vi "niFpgaButterflyTemp_2Pipe.vi"(0 "x_r":fxp<+/-,16,1>, 1 "mult output type":fxp<+/-,18,2>, 2 "bf bullet type":fxp<+/-,32,16> format="%.21g", 5 "x_i":fxp<+/-,16,1>, 7 "y_r":fxp<+/-,16,1>, 9 "y_i":fxp<+/-,16,1>, 12 "tf_r":fxp<+/-,16,1>, 13 "tf_i":fxp<+/-,16,1>, 14 "first stage":bool) -> (4 "x_out_r":fxp<+/-,16,1>, 6 "x_out_i":fxp<+/-,16,1>, 8 "y_out_r":fxp<+/-,16,1>, 10 "y_out_i":fxp<+/-,16,1>)   [LabVIEW 2017]
uses:
  <vilib>/rvi/FXPMathLib/FxpMul/XNode/nifxpmath_Multiplier.xnode
  <vilib>/rvi/FXPMathLib/sim/FxpSim.dll
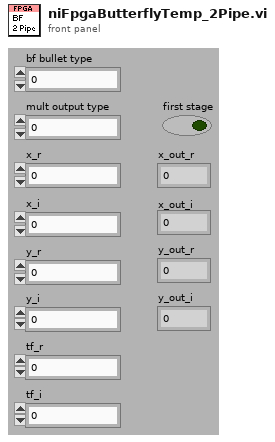
[diagram p1: front panel]
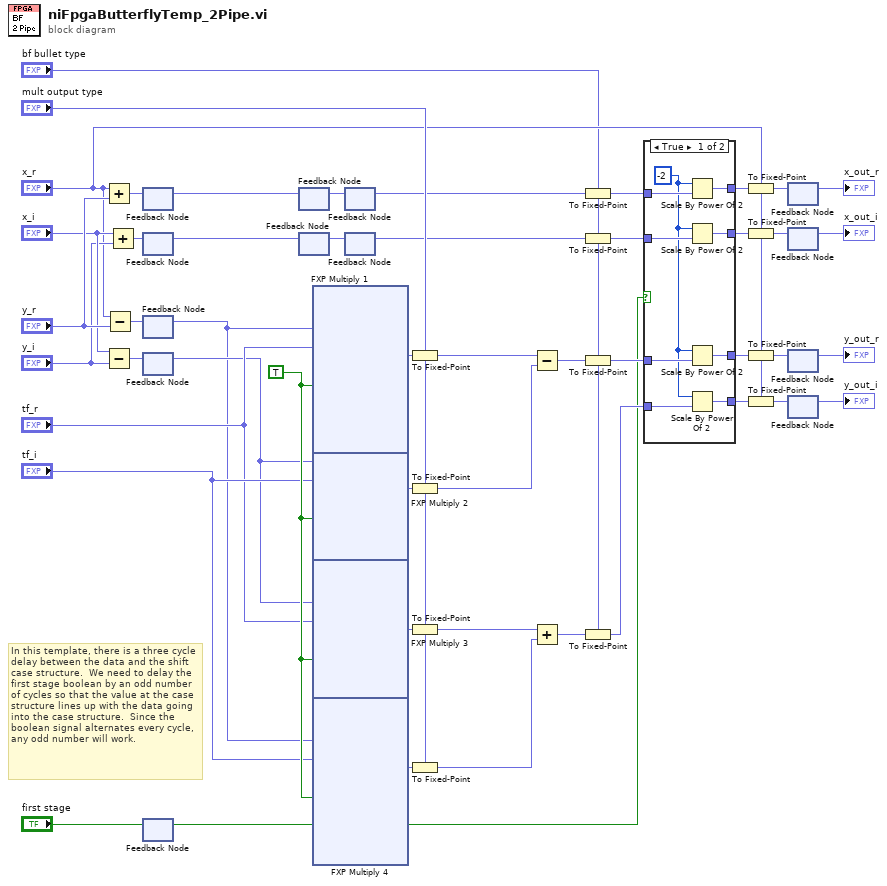
[diagram p0: block diagram]
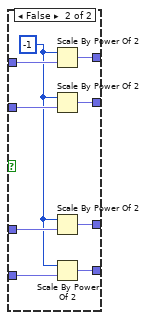
[diagram p2: hidden frame]
diagram:
  w40 = TRUE ("input valid")
  # "In this template, there is a three cycle delay between the data and the shift case structure.  We need to delay the first stage boolean by an odd number of cycles so that the value at the case structure lines up with the data going into the case structure.  Since the boolean signal alternates every cycle, any odd number will work."
  n1 = Add(x="x_r", y="y_r") -> (x+y=w37:fxp<+/-,17,2>)
  n2 = Subtract(x="x_i", y="y_i") -> (x-y=w48:fxp<+/-,17,2>)
  n3 = Subtract(x="x_r", y="y_r") -> (x-y=w49:fxp<+/-,17,2>)
  n4 = Add(x="x_i", y="y_i") -> (x+y=w16:fxp<+/-,17,2>)
  n5 = feedback-in #1(w37) -> ()
  n6 = feedback #1() -> (w20:fxp<+/-,17,2>)  [unwired: 1 out]
  n7 = feedback-in #2(w16) -> ()
  n8 = feedback #2() -> (w18:fxp<+/-,17,2>)  [unwired: 1 out]
  n9 = feedback-in #3(w49) -> ()
  n10 = feedback #3() -> (w14:fxp<+/-,17,2>)  [unwired: 1 out]
  n11 = feedback-in #4(w48) -> ()
  n12 = feedback #4() -> (w15:fxp<+/-,17,2>)  [unwired: 1 out]
  n13 = feedback-in #5("first stage") -> ()
  n14 = feedback #5() -> (w2:bool)  [unwired: 1 out]
  n15 = feedback-in #6(w20) -> ()
  n16 = feedback #6() -> (w19:fxp<+/-,17,2>)  [unwired: 1 out]
  n17 = feedback-in #7(w18) -> ()
  n18 = feedback #7() -> (w17:fxp<+/-,17,2>)  [unwired: 1 out]
  n19 = xnode "FXP Multiply 1"("x"=w14, "y"="tf_r", "input valid"=w40) -> ("x*y"=w3:fxp<+/-,33,3>)  [unwired: 1 in, 2 out]
  n20 = xnode "FXP Multiply 2"("x"=w15, "y"="tf_i", "input valid"=w40) -> ("x*y"=w32:fxp<+/-,33,3>)  [unwired: 1 in, 2 out]
  n21 = xnode "FXP Multiply 3"("x"=w15, "y"="tf_r", "input valid"=w40) -> ("x*y"=w34:fxp<+/-,33,3>)  [unwired: 1 in, 2 out]
  n22 = xnode "FXP Multiply 4"("x"=w14, "y"="tf_i", "input valid"=w40) -> ("x*y"=w36:fxp<+/-,33,3>)  [unwired: 1 in, 2 out]
  n23 = feedback-in #8(w19) -> ()
  n24 = feedback #8() -> (w13:fxp<+/-,17,2>)  [unwired: 1 out]
  n25 = feedback-in #9(w17) -> ()
  n26 = feedback #9() -> (w12:fxp<+/-,17,2>)  [unwired: 1 out]
  n27 = To Fixed-Point(fixed-point type="mult output type", number=w3) -> (fixed-point=w30:fxp<+/-,18,2>)
  n28 = To Fixed-Point(fixed-point type="mult output type", number=w32) -> (fixed-point=w31:fxp<+/-,18,2>)
  n29 = To Fixed-Point(fixed-point type="mult output type", number=w34) -> (fixed-point=w33:fxp<+/-,18,2>)
  n30 = To Fixed-Point(fixed-point type="mult output type", number=w36) -> (fixed-point=w35:fxp<+/-,18,2>)
  n31 = Subtract(x=w30, y=w31) -> (x-y=w25:fxp<+/-,19,3>)
  n32 = Add(x=w33, y=w35) -> (x+y=w27:fxp<+/-,19,3>)
  n33 = To Fixed-Point(fixed-point type="bf bullet type", number=w13) -> (fixed-point=w23:fxp<+/-,32,16>)
  n34 = To Fixed-Point(fixed-point type="bf bullet type", number=w12) -> (fixed-point=w22:fxp<+/-,32,16>)
  n35 = To Fixed-Point(fixed-point type="bf bullet type", number=w25) -> (fixed-point=w24:fxp<+/-,32,16>)
  n36 = To Fixed-Point(fixed-point type="bf bullet type", number=w27) -> (fixed-point=w26:fxp<+/-,32,16>)
  n37 = case shown="True" w2 {
    tunnel: [w58 w67] -> w44
    tunnel: [w57 w66] -> w43
    tunnel: [w56 w65] -> w42
    tunnel: [w55 w64] -> w41
    tunnel: w26 -> [w54 w63]
    tunnel: w24 -> [w53 w62]
    tunnel: w23 -> [w52 w61]
    tunnel: w22 -> [w51 w60]
    frame True {
      w50 = -2 ("n")
      n38 = Scale By Power Of 2(n=w50, x=w52) -> (x*2^n=w58:fxp<+/-,32,16>)
      n39 = Scale By Power Of 2(n=w50, x=w51) -> (x*2^n=w57:fxp<+/-,32,16>)
      n40 = Scale By Power Of 2(n=w50, x=w53) -> (x*2^n=w56:fxp<+/-,32,16>)
      n41 = Scale By Power Of 2(n=w50, x=w54) -> (x*2^n=w55:fxp<+/-,32,16>)
    }
    frame False {
      w59 = -1 ("n")
      n42 = Scale By Power Of 2(n=w59, x=w61) -> (x*2^n=w67:fxp<+/-,32,16>)
      n43 = Scale By Power Of 2(n=w59, x=w60) -> (x*2^n=w66:fxp<+/-,32,16>)
      n44 = Scale By Power Of 2(n=w59, x=w62) -> (x*2^n=w65:fxp<+/-,32,16>)
      n45 = Scale By Power Of 2(n=w59, x=w63) -> (x*2^n=w64:fxp<+/-,32,16>)
    }
  }
  n46 = To Fixed-Point(fixed-point type="x_r", number=w44) -> (fixed-point=w10:fxp<+/-,16,1>)
  n47 = To Fixed-Point(fixed-point type="x_r", number=w43) -> (fixed-point=w11:fxp<+/-,16,1>)
  n48 = To Fixed-Point(fixed-point type="x_r", number=w42) -> (fixed-point=w9:fxp<+/-,16,1>)
  n49 = To Fixed-Point(fixed-point type="x_r", number=w41) -> (fixed-point=w8:fxp<+/-,16,1>)
  n50 = feedback-in #10(w10) -> ()
  n51 = feedback #10() -> (→"x_out_r":fxp<+/-,16,1>)  [unwired: 1 out]
  n52 = feedback-in #11(w11) -> ()
  n53 = feedback #11() -> (→"x_out_i":fxp<+/-,16,1>)  [unwired: 1 out]
  n54 = feedback-in #12(w9) -> ()
  n55 = feedback #12() -> (→"y_out_r":fxp<+/-,16,1>)  [unwired: 1 out]
  n56 = feedback-in #13(w8) -> ()
  n57 = feedback #13() -> (→"y_out_i":fxp<+/-,16,1>)  [unwired: 1 out]
